vi "Get Class Functions C Description.vi"(8 "error in (no error)":errorcluster, 10 "Access Scope":T1(ring)=enum."public", 11 "LabVIEW Obj":refnum<class>) -> (0 "error out":errorcluster, 3 "Array":string[](array[string]))   [LabVIEW 2017]
uses:
  String/Strip Class Function Name.vi/82d5ef48-2c95-4ac8-8452-541d4ca00c93.vi
  String/Strip Class Function Name.vi/8c0b350f-6b41-4dd8-8255-dad520baa4a5.vi
  <vilib>/Utility/VariantDataType/VariantType.lvlib
  _openG/_reuse_openG.lvlib
  <vilib>/Utility/Data Type/NI_Data Type.lvlib
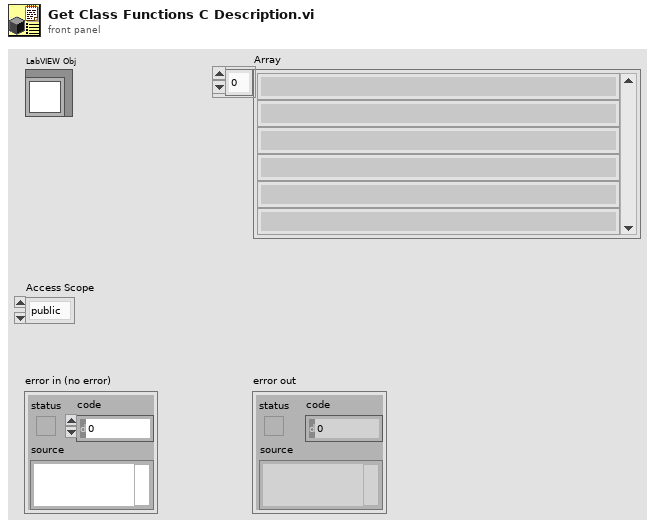
[diagram p1: front panel]
types:
  T1 = enum32{"invalid scope", "public", "private", "protected", "community"}
  T2 = typedef "VariantType.lvlib/VIInfo.ctl" = cluster{"Data1":i16, "Data2":i16, "Flags":u32[], "Modification Date":timestamp, "Asynchronous":bool, "NonFunctional":bool, "Subroutine":bool, "SubSystem":bool}
  T3 = typedef "NI_Data Type.lvlib/Data Type.ctl" = enum8{"Invalid Type", "Void", "I8", "I16", "I32", "I64", "U8", "U16", "U32", "U64", "Single Float", "Double Float", "Extended Float", "Single Complex", "Double Complex", "Extended Complex", "Enum U8", "Enum U16", "Enum U32", "Enum U64", "Single Float With Unit", "Double Float With Unit", "Extended Float With Unit", "Single Complex with Unit", "Double Complex with Unit", "Extended Complex with Unit", "Boolean", "String", "Path", "Picture", "Tag", "Array", "Cluster", "Variant", "LV Variant", "Waveform", "Timestamp", "Digital Waveform", "Digital Data", "ExpressData", "Refnum", "External Data", "VI", "Poly VI", "LabVIEW Class Instance", "Fixed Point"}
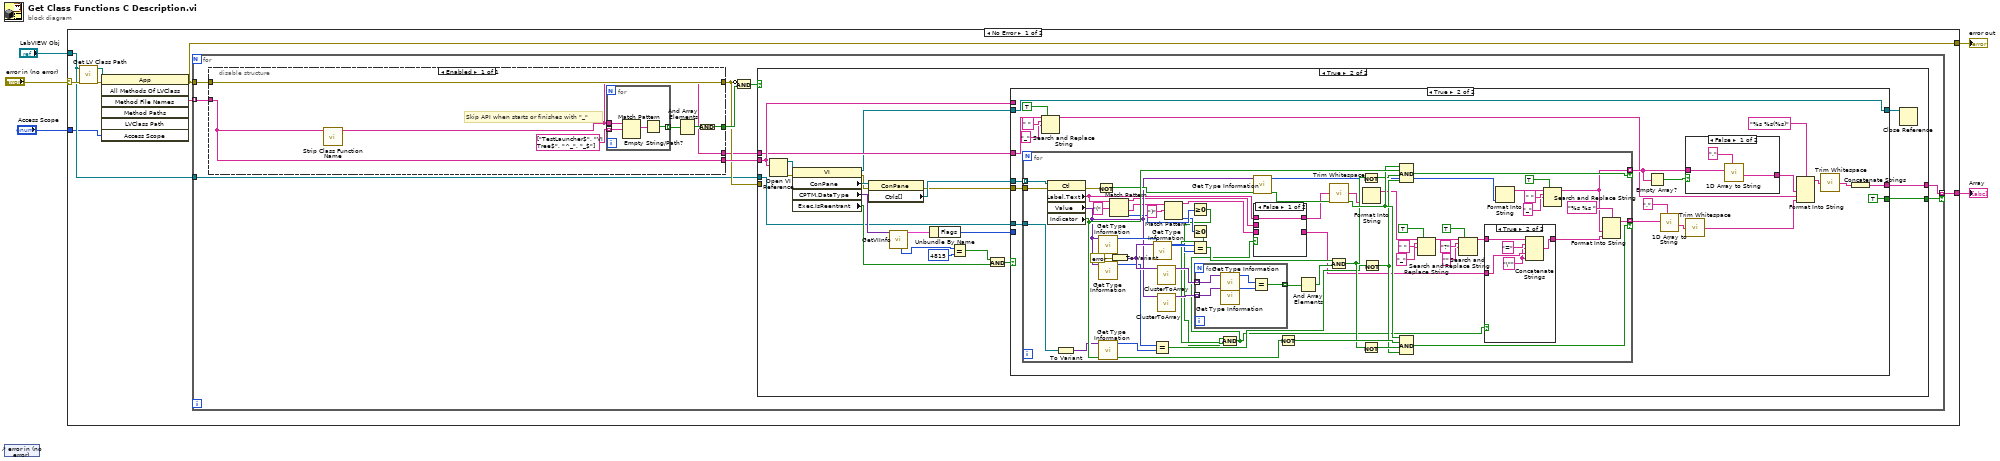
[diagram p0: block diagram]
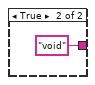
[diagram p4: hidden frame]
diagram:
  n1 = control-ref of="error in (no error)"() -> ()  [unwired: 1 out]
  n2 = case shown="No Error" "error in (no error)" {
    selector: "error in (no error)" -> [w12 w155]
    tunnel: [w9 w155] -> w4
    tunnel: "LabVIEW Obj" -> [w7 _]
    tunnel: [w8 _] -> w2
    tunnel: "Access Scope" -> [w6 _]
    frame No Error {
      n3 = call <vilib>:"Get LV Class Path.vi"("error in (no error)"=w12, "object"=w7) -> ("error out"=w10:errorcluster, "class path"=w13:path)  [unwired: 8 in]
      n4 = invoke class="App" method="All Methods Of LVClass"(error in=w10, "LVClass Path"=w13, "Access Scope"=w6) -> (error out=w9:errorcluster, "Method File Names"=w11:string[])  [unwired: 4 in, 5 out]
      n5 = for {
        tunnel: w11 -> [w19] mode=indexing
        tunnel: [w23] -> w8 mode=indexing if=w22
        tunnel: w9 -> [w20]
        tunnel: w7 -> [w14]
        n6 = disable-structure shown="Enabled" {
          disable-tunnel: [w24] -> w21
          disable-tunnel: w20 -> [w27]
          disable-tunnel: w19 -> [w24]
          disable-tunnel: [w26] -> w18
          disable-tunnel: [w27] -> w16
          disable-tunnel: [w25] -> w15
          frame Enabled {
            # "Skip API when starts or finishes with \"_\""
            n7 = call "Strip Class Function Name.vi"("File Full Path Name"=w24) -> ("Function Name"=w25:string)  [unwired: 2 in, 2 out]
            n8 = for {
              tunnel: w25 -> [w34]
              tunnel: string[] ["TestLauncher$", "VI Tree$", "^_", "_$"] -> [w33] mode=indexing
              tunnel: [w31] -> w28 mode=indexing
              n9 = Match Pattern(string=w34, regular expression=w33) -> (match substring=w32:string)  [unwired: 1 in, 3 out]
              n10 = Empty String/Path?(string/path=w32) -> (empty?=w31:bool)
            }
            n11 = And Array Elements(Boolean array=w28) -> (logical AND=w30:bool)
            n12 = Compound Arithmetic op=AND(w30) -> (w26:bool)
          }
        }
        n13 = Compound Arithmetic op=AND(invert w16, w18) -> (w17:bool)
        n14 = case shown="True" w17 {
          tunnel: [_ w55] -> w23
          tunnel: [_ w54] -> w22
          tunnel: w21 -> [_ w53]
          tunnel: w16 -> [_ _]
          tunnel: w15 -> [_ w52]
          tunnel: w14 -> [_ w35]
          frame False {
          }
          frame True {
            n15 = Open VI Reference(vi path=w53) -> (vi reference=w47:refnum<vi>, error out=w48:errorcluster)  [unwired: 5 in]
            n16 = property class="VI"(reference=w47, error in=w48) -> (reference out=w38:refnum<vi>, error out=w46:errorcluster, "ConPane"=w51:refnum<vi>, "CPTM.DataType"=w45:variant, "Exec.IsReentrant"=w39:bool)
            n17 = property class="ConPane"(reference=w51, error in=w46) -> (error out=w36:errorcluster, "Ctrls[]"=w50:refnum<vi>[])  [unwired: 1 out]
            n18 = call <vilib>:"GetVIInfo.vi"("Variant"=w45) -> ("VI Info"=w43:T2, "pattern"=w44:i16)  [unwired: 6 in, 3 out]
            n19 = Unbundle By Name(w43) -> ("Flags"=w42:u32[])
            n20 = Equal?(x=w44, y=i16 4815) -> (x = y?=w41:bool)
            n21 = Compound Arithmetic op=AND(w41, w39) -> (w40:bool)
            n22 = case shown="True" w40 {
              tunnel: [_ w57] -> w55
              tunnel: w50 -> [_ w76]
              tunnel: [_ TRUE] -> w54
              tunnel: w53 -> [_ _]
              tunnel: w52 -> [_ w61]
              tunnel: w42 -> [_ _]
              tunnel: w38 -> [w56 w77]
              tunnel: [w56 w77] -> w37
              tunnel: w36 -> [_ w69]
              tunnel: w35 -> [_ w67]
              frame False {
              }
              frame True {
                n23 = for {
                  tunnel: w76 -> [w140] mode=indexing
                  tunnel: [w102] -> w66 mode=indexing if=w133
                  tunnel: [w138] -> w74 mode=indexing if=w132
                  tunnel: w69 -> [w135]
                  tunnel: w67 -> [w116]
                  n24 = property class="Ctl"(reference=w140, error in=w135) -> (error out=w134:errorcluster, "Label.Text"=w95:string, "Value"=w115:variant, "Indicator"=w137:bool)  [unwired: 1 out]
                  n25 = To Variant(anything=w116) -> (Variant=w117:variant)
                  n26 = Not(x=w134) -> (.not. x?=w131:bool)
                  n27 = call <vilib>:"Get Type Information.vi"("Variant"=w115) -> ("Type"=w129:T3)  [unwired: 6 in, 4 out]
                  n28 = call <vilib>:"Get Type Information.vi"("Variant"=w115) -> ("Type"=w114:T3)  [unwired: 6 in, 4 out]
                  n29 = call <vilib>:"Get Type Information.vi"("Variant"=w117) -> ("Type"=w113:T3)  [unwired: 6 in, 4 out]
                  n30 = Match Pattern(string=w95, regular expression="(") -> (before substring=w93:string, after substring=w88:string, offset past match=w99:i32)  [unwired: 1 in, 1 out]
                  n31 = To Variant(anything=errorcluster {"status"=FALSE, "code"=0, "source"=""} ("error in (no error)")) -> (Variant=w127:variant)
                  n32 = call <vilib>:"Get Type Information.vi"("Variant"=w127) -> ("Type"=w128:T3)  [unwired: 6 in, 4 out]
                  n33 = Equal?(x=w114, y=w113) -> (x = y?=w112:bool)
                  n34 = call "ClusterToArray.vi"("Cluster"=w127) -> ("Array"=w126:variant[])  [unwired: 9 in, 1 out]
                  n35 = call "ClusterToArray.vi"("Cluster"=w115) -> ("Array"=w125:variant[])  [unwired: 9 in, 1 out]
                  n36 = Match Pattern(string=w88, regular expression=")") -> (before substring=w89:string, offset past match=w98:i32)  [unwired: 1 in, 2 out]
                  n37 = Greater Or Equal To 0?(x=w99) -> (x >= 0?=w96:bool)
                  n38 = Greater Or Equal To 0?(x=w98) -> (x >= 0?=w97:bool)
                  n39 = Equal?(x=w129, y=w128) -> (x = y?=w124:bool)
                  n40 = for {
                    tunnel: w126 -> [w154] mode=indexing
                    tunnel: w125 -> [w153] mode=indexing
                    tunnel: [w150] -> w123 mode=indexing
                    n41 = call <vilib>:"Get Type Information.vi"("Variant"=w154) -> ("Type"=w152:T3)  [unwired: 6 in, 4 out]
                    n42 = call <vilib>:"Get Type Information.vi"("Variant"=w153) -> ("Type"=w151:T3)  [unwired: 6 in, 4 out]
                    n43 = Equal?(x=w152, y=w151) -> (x = y?=w150:bool)
                  }
                  n44 = And(x=w96, y=w97) -> (x .and. y?=w92:bool)
                  n45 = call <vilib>:"Get Type Information.vi"("Variant"=w115) -> ("Type"=w118:T3)  [unwired: 6 in, 4 out]
                  n46 = case shown="False" w92 {
                    tunnel: [w147 w149] -> w94
                    tunnel: w95 -> [w147 _]
                    tunnel: w93 -> [_ w149]
                    tunnel: [_ w148] -> w90
                    tunnel: w89 -> [_ w148]
                    frame False {
                    }
                    frame True {
                    }
                  }
                  n47 = Not(x=w137) -> (.not. x?=w136:bool)
                  n48 = And Array Elements(Boolean array=w123) -> (logical AND=w121:bool)
                  n49 = call <vilib>:"Trim Whitespace.vi"("string"=w94) -> ("trimmed string"=w87:string)  [unwired: 1 in]
                  n50 = Compound Arithmetic op=AND(w124, w121) -> (w122:bool)
                  n51 = Not(x=w122) -> (.not. x?=w119:bool)
                  n52 = Not(x=w122) -> (.not. x?=w120:bool)
                  n53 = Format Into String(w87) -> (resulting string=w103:string)  [unwired: 3 in, 1 out]
                  n54 = Not(x=w112) -> (.not. x?=w111:bool)
                  n55 = Compound Arithmetic op=AND(w131, w137, w119, w111) -> (w133:bool)
                  n56 = Compound Arithmetic op=AND(w131, w136, w120, w111) -> (w132:bool)
                  n57 = Search and Replace String(replace all?=TRUE ("replace all? (F)"), input string=w103, search string=" ", replace string="_" ("replace string (\"\")")) -> (result string=w83:string)  [unwired: 4 in, 3 out]
                  n58 = Search and Replace String(replace all?=TRUE ("replace all? (F)"), input string=w83, search string="?", replace string="" ("replace string (\"\")")) -> (result string=w82:string)  [unwired: 4 in, 3 out]
                  n59 = case shown="True" w92 {
                    tunnel: w82 -> [w141 w145]
                    tunnel: [w141 w146] -> w91
                    tunnel: w90 -> [_ w143]
                    frame False {
                    }
                    frame True {
                      w142 = "\"" ("string")
                      n60 = Concatenate Strings(w145, "=" ("string"), w142, w143, w142) -> (w146:string)
                    }
                  }
                  n61 = Format Into String(w118) -> (resulting string=w110:string)  [unwired: 3 in, 1 out]
                  n62 = Search and Replace String(replace all?=TRUE ("replace all? (F)"), input string=w110, search string=" ", replace string="_" ("replace string (\"\")")) -> (result string=w102:string)  [unwired: 4 in, 3 out]
                  n63 = Format Into String(format string="%s %s ", w102, w91) -> (resulting string=w138:string)  [unwired: 2 in, 1 out]
                }
                n64 = Search and Replace String(replace all?=TRUE ("replace all? (F)"), input string=w61, search string=" ", replace string="_" ("replace string (\"\")")) -> (result string=w60:string)  [unwired: 4 in, 3 out]
                n65 = Empty Array?(array=w66) -> (empty?=w65:bool)
                n66 = call "1D Array to String.vi"("delimiter (Tab)"=",", "Array of Strings"=w74) -> ("delimited string"=w71:string)  [unwired: 9 in]
                n67 = case shown="False" w65 {
                  tunnel: [w79 "void" ("delimited string")] -> w72
                  tunnel: w66 -> [w78 _]
                  frame False {
                    n68 = call "1D Array to String.vi"("delimiter (Tab)"=",", "Array of Strings"=w78) -> ("delimited string"=w79:string)  [unwired: 9 in]
                  }
                  frame True {
                  }
                }
                n69 = call <vilib>:"Trim Whitespace.vi"("string"=w71) -> ("trimmed string"=w58:string)  [unwired: 1 in]
                n70 = Format Into String(format string="%s %s(%s)", w72, w60, w58) -> (resulting string=w70:string)  [unwired: 2 in, 1 out]
                n71 = call <vilib>:"Trim Whitespace.vi"("string"=w70) -> ("trimmed string"=w59:string)  [unwired: 1 in]
                n72 = Concatenate Strings(w59) -> (w57:string)
              }
            }
            n73 = Close Reference(reference=w37) -> ()  [unwired: 1 in, 1 out]
          }
        }
      }
    }
    frame Error {
    }
  }
  "error out" <- w4
  "Array" <- w2
